vi "行插入.vi"(8 "error in (no error)":errorcluster caption="错误输入（无错误）", 11 "程序 输入":refnum<class "程序.lvclass">) -> (0 "error out":errorcluster caption="错误输出", 3 "程序 输出":refnum<class "程序.lvclass">)   [LabVIEW 2020, in "程序.lvclass"]
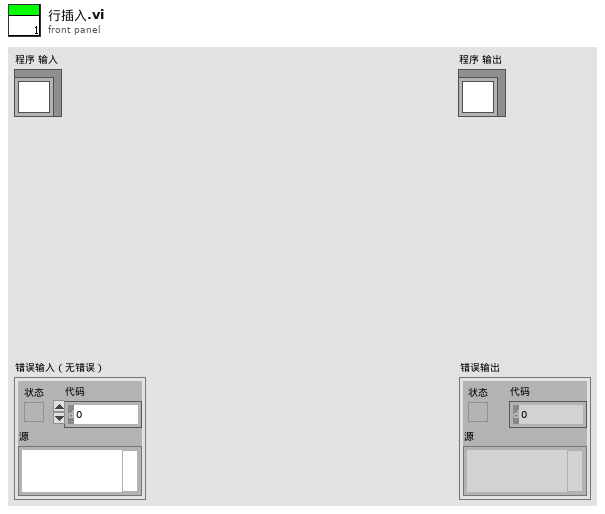
[diagram p1: front panel]
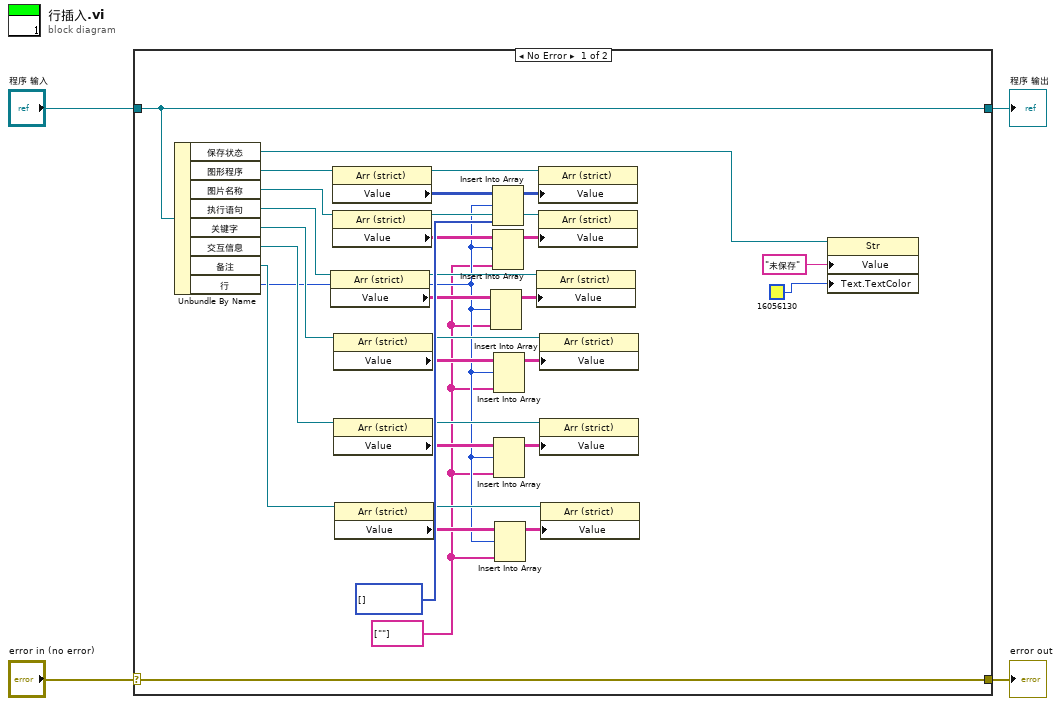
[diagram p0: block diagram]
diagram:
  n1 = case shown="No Error" "error in (no error)" {
    selector: "error in (no error)" -> [w36 w38]
    tunnel: [w36 w38] -> w3
    tunnel: [w35 w37] -> w1
    tunnel: "程序 输入" -> [w35 w37]
    frame No Error {
      w5 = string[] [""] ("新元素/子数组")
      n2 = Unbundle By Name(w35) -> ("保存状态"=w11:refnum<vi>, "图形程序"=w34:refnum<vi>, "图片名称"=w26:refnum<vi>, "执行语句"=w22:refnum<vi>, "关键字"=w19:refnum<vi>, "交互信息"=w14:refnum<vi>, "备注"=w7:refnum<vi>, "行"=w6:u32)
      n3 = property class="Arr (strict)"(reference=w22) -> (reference out=w23:refnum<vi>, "Value"=w24:string[][])  [unwired: 1 in, 1 out]
      n4 = property class="Arr (strict)"(reference=w34) -> (reference out=w33:refnum<vi>, "Value"=w32:picture[][])  [unwired: 1 in, 1 out]
      n5 = property class="Arr (strict)"(reference=w26) -> (reference out=w27:refnum<vi>, "Value"=w28:string[][])  [unwired: 1 in, 1 out]
      n6 = property class="Arr (strict)"(reference=w19) -> (reference out=w18:refnum<vi>, "Value"=w21:string[][])  [unwired: 1 in, 1 out]
      n7 = property class="Arr (strict)"(reference=w14) -> (reference out=w15:refnum<vi>, "Value"=w16:string[][])  [unwired: 1 in, 1 out]
      n8 = property class="Arr (strict)"(reference=w7) -> (reference out=w10:refnum<vi>, "Value"=w9:string[][])  [unwired: 1 in, 1 out]
      n9 = Insert Into Array(array=w24, index (row)=w6, new element=w5) -> (w25:string[][])  [unwired: 1 in]
      n10 = Insert Into Array(array=w32, index (row)=w6, new element=picture[] [] ("新元素/子数组")) -> (w31:picture[][])  [unwired: 1 in]
      n11 = Insert Into Array(array=w28, index (row)=w6, new element=w5) -> (w29:string[][])  [unwired: 1 in]
      n12 = Insert Into Array(array=w21, index (row)=w6, new element=w5) -> (w20:string[][])  [unwired: 1 in]
      n13 = Insert Into Array(array=w16, index (row)=w6, new element=w5) -> (w17:string[][])  [unwired: 1 in]
      n14 = Insert Into Array(array=w9, index (row)=w6, new element=w5) -> (w8:string[][])  [unwired: 1 in]
      n15 = property class="Arr (strict)"(reference=w23, "Value"=w25) -> ()  [unwired: 1 in, 2 out]
      n16 = property class="Arr (strict)"(reference=w33, "Value"=w31) -> ()  [unwired: 1 in, 2 out]
      n17 = property class="Arr (strict)"(reference=w27, "Value"=w29) -> ()  [unwired: 1 in, 2 out]
      n18 = property class="Arr (strict)"(reference=w18, "Value"=w20) -> ()  [unwired: 1 in, 2 out]
      n19 = property class="Arr (strict)"(reference=w15, "Value"=w17) -> ()  [unwired: 1 in, 2 out]
      n20 = property class="Arr (strict)"(reference=w10, "Value"=w8) -> ()  [unwired: 1 in, 2 out]
      n21 = property class="Str"(reference=w11, "Value"="未保存" ("值"), "Text.TextColor"=u32 16056130) -> ()  [unwired: 1 in, 2 out]
    }
    frame Error {
    }
  }
  "error out" <- w3
  "程序 输出" <- w1
